vi "CliGetProtection.vi"(0 "ref in":u64, 11 "error in (no error)":errorcluster) -> (1 "sch_schal":u16, 2 "sch_par":u16, 3 "sch_rel":u16, 4 "ref out":u64, 6 "Result":i32, 13 "bart_sch":u16, 14 "anl_sch":u16, 15 "error out":errorcluster)   [LabVIEW 2020, in "Snap7.lvlib"]
uses:
  Snap7.lvlib
  windows/lv_snap7.dll
panel:
  in  "var protection":T1
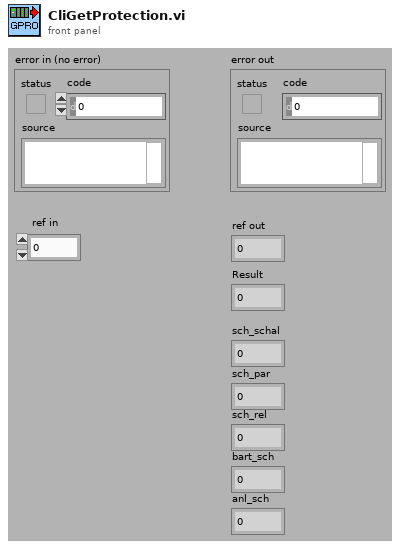
[diagram p1: front panel]
types:
  T1 = cluster{"sch_schal":u16, "sch_par":u16, "sch_rel":u16, "bart_sch":u16, "anl_sch":u16}
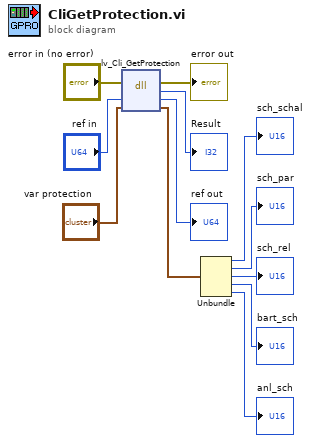
[diagram p0: block diagram]
diagram:
  n1 = dll-call lib="PTH2iabs CUsersFeng项目HLCEPS300-1老性能试验台SourcesSnap7libwindowslv_snap7.dll" fn="lv_Cli_GetProtection"(error in="error in (no error)", "Client"="ref in", "var_Info"="var protection") -> (error out=→"error out":errorcluster, "return type"=→"Result":i32, "Client"=→"ref out":u64, "var_Info"=w7:T1)  [unwired: 2 in, 1 out]
  n2 = Unbundle(w7) -> ("sch_schal"=→"sch_schal":u16, "sch_par"=→"sch_par":u16, "sch_rel"=→"sch_rel":u16, "bart_sch"=→"bart_sch":u16, "anl_sch"=→"anl_sch":u16)
